vi "Multiply Force.vi"(10 "force in":dbl, 11 "Pounding Tool":refnum<class "Pounding Tool.lvclass">) -> (2 "force out":dbl)   [LabVIEW 2023, in "Pounding Tool.lvclass"]
uses:
  Pounding Tool.lvclass
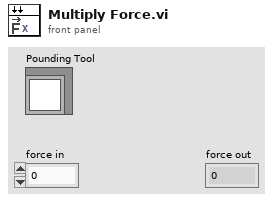
[diagram p1: front panel]
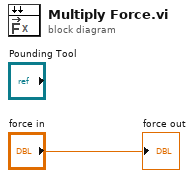
[diagram p0: block diagram]
diagram:
  "force out" <- "force in"
